vi "Save Settings.vi"(8 "error in (no error)":errorcluster, 9 "Section":string, 10 "Path":path, 11 "Save Restore Settings in":refnum<class "Save Restore Settings.lvclass">) -> (0 "error out":errorcluster, 3 "Save Restore Settings out":refnum<class "Save Restore Settings.lvclass">)   [LabVIEW 2020, in "Save Restore Settings.lvclass"]
uses:
  <userlib>/_MGI/Application Control/MGI Save Restore Settings/Save Restore Settings.lvclass
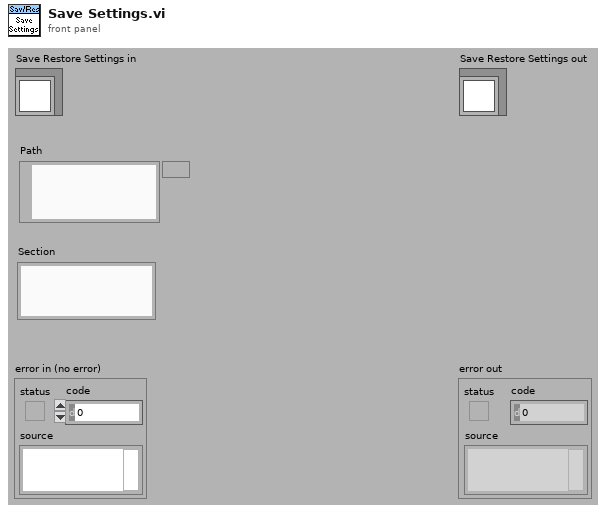
[diagram p1: front panel]
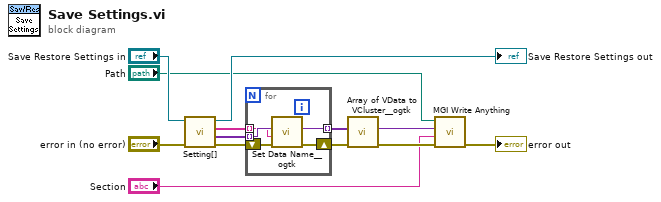
[diagram p0: block diagram]
diagram:
  n1 = call-dynamic "Setting[].vi"("error in (no error)"="error in (no error)", "Save Restore Settings in"="Save Restore Settings in") -> ("error out"=w7:errorcluster, "Value[]"=w6:variant[], "Tag[]"=w5:string[], "Save Restore Settings out"=→"Save Restore Settings out":refnum<class "Save Restore Settings.lvclass">)  [unwired: 6 in]
  n2 = for {
    shift-right: [w15] -> w3
    shift-left: w7 -> [w18]
    tunnel: w6 -> [w17] mode=indexing
    tunnel: w5 -> [w16] mode=indexing
    tunnel: [w14] -> w4 mode=indexing
    n3 = call <userlib>:"Set Data Name__ogtk.vi"("error in (no error)"=w18, "Data Name"=w16, "Data"=w17) -> ("error out"=w15:errorcluster, "Renamed Data"=w14:variant)  [unwired: 7 in]
  }
  n4 = call <userlib>:"Array of VData to VCluster__ogtk.vi"("error in (no error)"=w3, "Array"=w4) -> ("error out"=w10:errorcluster, "VCluster"=w2:variant)  [unwired: 8 in]
  n5 = call <userlib>:"MGI Write Anything.vi"("Error In"=w10, "Section Name (Name of \"Anything\")"="Section", "Anything"=w2, "Path (dialog)"="Path") -> ("Error Out"=→"error out":errorcluster)  [unwired: 5 in, 2 out]
